vi "CTRE_CANifier_GetPWMInput.vi"(8 "error in":errorcluster, 10 "PWMChannel":T1, 11 "CANifierDevRef":T2) -> (0 "error out":errorcluster, 1 "Period":sgl, 2 "Duty Cycle":sgl, 3 "CANifierDevRef":T2)   [LabVIEW 2020]
uses:
  <vilib>/Rock Robotics/WPI/ThirdParty/Phoenix-LabVIEW/CANifier/CTRE_CANifier_DeviceRef.ctl
  <vilib>/Rock Robotics/WPI/ThirdParty/Phoenix-LabVIEW/CANifier/CTRE_CANifier_PWMChannel.ctl
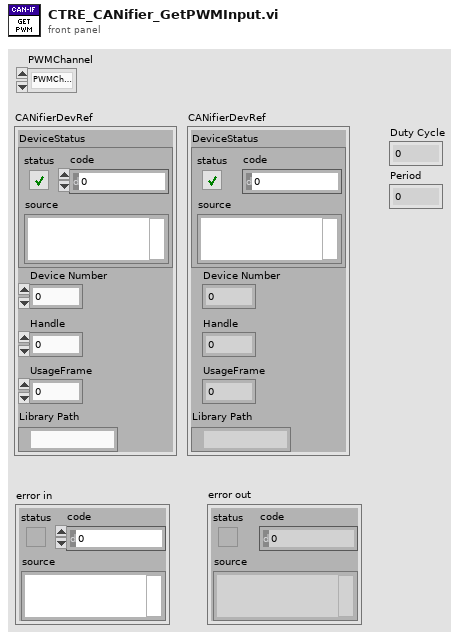
[diagram p1: front panel]
types:
  T1 = typedef "CTRE_CANifier_PWMChannel.ctl" = enum16{"PWMChannel0", "PWMChannel1", "PWMChannel2", "PWMChannel3"}
  T2 = typedef "CTRE_CANifier_DeviceRef.ctl" = cluster{"DeviceStatus":errorcluster, "Device Number":u8, "Handle":u64, "UsageFrame":u32, "Library Path":path}
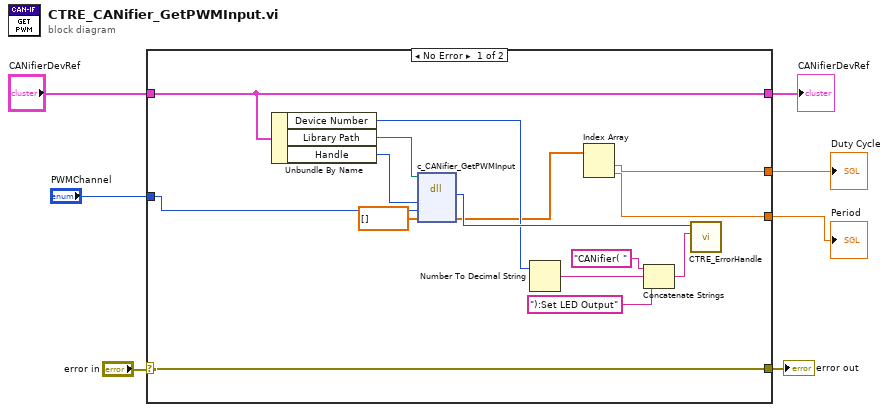
[diagram p0: block diagram]
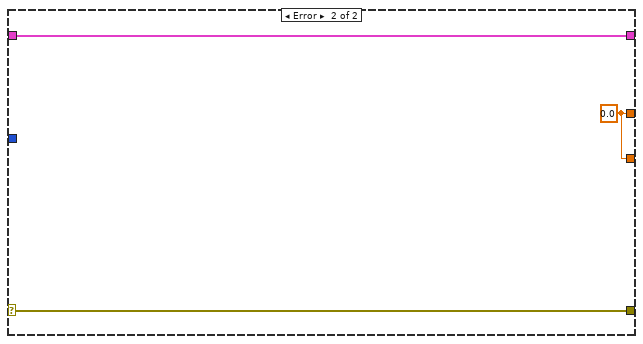
[diagram p2: hidden frame]
diagram:
  n1 = case shown="No Error" "error in" {
    selector: "error in" -> [w22 w25]
    tunnel: [w22 w25] -> w6
    tunnel: "CANifierDevRef" -> [w21 w24]
    tunnel: [w21 w24] -> w4
    tunnel: "PWMChannel" -> [w12 _]
    tunnel: [w10 w23] -> w2
    tunnel: [w9 w23] -> w1
    frame No Error {
      n2 = Unbundle By Name(w21) -> ("Device Number"=w14:u8, "Library Path"=w20:path, "Handle"=w19:u64)
      n3 = dll-call lib="?" fn="c_CANifier_GetPWMInput"(path in=w20, "handle"=w19, "pwmChannel"=w12, "dutyCycleAndPeriod"=dbl[] []) -> ("CTR_Code"=w18:i8, "dutyCycleAndPeriod"=w11:dbl[])  [unwired: 4 in, 2 out]
      n4 = Number To Decimal String(number=w14) -> (decimal integer string=w17:string)  [unwired: 1 in]
      n5 = Index Array(array=w11) -> (element #1=w10:dbl, element #2=w9:dbl)  [unwired: 2 in]
      n6 = Concatenate Strings("CANifier( " ("string"), w17, "):Set LED Output" ("string")) -> (w13:string)
      n7 = call <vilib>:"CTRE_ErrorHandle.vi"("origin"=w13, "code"=w18) -> ()  [unwired: 9 in, 1 out]
    }
    frame Error {
      w23 = sgl 0.0
    }
  }
  "error out" <- w6
  "CANifierDevRef" <- w4
  "Duty Cycle" <- w2
  "Period" <- w1
